vi "Fetch Multiple Records_20230203.vi"(0 "device session in":refnum<class "Device Session.lvclass">, 1 "starting record":u64, 2 "number of records":u64=1, 3 "Chan#":T1=enum."1", 5 "fetch relative to":T2=enum."First Pretrigger Sample", 7 "number of samples":u64=1000, 9 "timeout (ms)":i32=1000, 11 "error in":errorcluster, 12 "fetch offset":i64) -> (4 "device session out":refnum<class "Device Session.lvclass">, 6 "data":dbl[][](array[numeric]), 8 "relativeX (samples)":dbl[](array[numeric]), 14 "requested records info":T3[](array[typedef]), 15 "error out":errorcluster)   [LabVIEW 2021, in "Device Session.lvclass"]
doc: "Fetches data from multiple records in an acquisition. No data is returned if this VI times out. You must run the <B>Initiate</B> VI before running this VI.\n\n<B>Input Parameters</B>\n\n<B>device session in</B> is a reference to the Device Session object, which contains a session to each instrument design library used in this sample project. This parameter is obtained from the 'Open Session' VI.\n\n<B>number of records</B> specifies the number of records to fetch samples from. The default value is 1.\n\n<B>starting record</B> specifies the record to retrieve. Index of the record numbers starts at 0.\n\n<B>fetch relative to</B> specifies the relative location within the acquired record from where the VI begins to fetch data.\n\n'First Sample': the fetch starts at the first sample acquired by the device. If the device wraps data in its memory buffer, the first sample is no longer available. In this case, the VI returns an error if 'fetch offset' specifies a location that is within the overwritten portion of the memory buffer.\n'Reference Trigger Sample': the fetch starts relative to the Reference Trigger.\n'First Pretrigger Sample': the fetch starts relative to the first pretrigger sample acquired. If you do not configure a Reference Trigger, 'First Pretrigger Sample' behaves the same as 'First Sample' because there are no pretrigger samples.\n'Most Recent Sample': the fetch starts relative to the most recently acquired sample. The value of 'fetch offset' must be negative. This VI doesn't support this option. Consider using the 'Fetch Single Record' VI instead.\n'Current Read Position': the fetch starts after the last fetched sample. This VI doesn't support this option. Consider using the 'Fetch Single Record' VI instead.\n\n<B>number of samples</B> specifies the number of samples to fetch. The default value is 1000.\n\n<B>timeout (ms)</B> specifies the time, in milliseconds, allotted for the Fetch Multiple Records VI to complete execution of each record before returning a timeout error. A value of -1 specifies that the VI waits until all data is available. A value of 0 is not supported. The default value is 10,000. You cannot abort a pending fetch using the Abort VI or Close VI.\n\n<B>fetch offset</B> specifies the offset relative to the position, which is specified by the 'fetch relative to' parameter, from which to start fetching data. Offset can be a positive or negative value. The default value is 0.\n\n<B>error in</B> describes error conditions that occur before this node runs. This input provides standard 'error in' functionality.\n\n<B>Output Parameters</B>\n\n<B>device session out</B> passes a reference to the session to the next VI.\n\n<B>data</B> returns the acquired records. Each waveform corresponds to a record. If the fetch contains multiple channels, all waveforms for a record are returned before proceeding to the next record. For example, a two-channel, two-record acquisition returns four waveforms:\narray index 0 = Channel0 Record0\narray index 1 = Channel1 Record0\narray index 2 = Channel0 Record1\narray index 3 = Channel1 Record1\n\n<B>relativeX (samples)</B> returns the relative positions from the trigger to the first sample in the acquired data.\n\n<B>requested records info</B> returns additional information about each record returned by 'data'. There is one element in the 'requested records info' array for each record.\n\n<B>requested records info.number of samples</B> returns the number of samples in the record.\n\n<B>requested records info.starting sample number</B> returns the sample number of the first sample in the returned record data. Sample numbers are zero-based. Sample numbers start at zero for each record and increment by one for each acquired sample.\n\n<B>requested records info.number of channels</B> returns the number of channels in the record data.\n\n<B>requested records info.timestamps</B> returns the timestamp values that were captured for the record.\n\n<B>error out</B> contains error information. This output provides standard 'error out' functionality."
uses:
  Device Session.lvclass
  <instrlib>/_niInstr/Multirecord Acquisition/Interface/v1/Host/Public/Requested Record Info.ctl
  <instrlib>/_niInstr/Multirecord Acquisition/Interface/v1/Host/Public/Fetch Relative To Enum.ctl
  Enums/Channel Numbers.ctl
  Device Session.lvclass/Device Session.ctl
  <instrlib>/_niInstr/Multirecord Acquisition/Interface/v1/Host/Private/Fetch Multiple Records DBL Wrapper.vi
  <instrlib>/HSAI-RIO/Config/Group A/v1/Host/Main/niHSAI Group A Config v1 Host.lvclass
  <instrlib>/_niInstr/Multirecord Acquisition/Interface/v1/Host/niInstr Multirecord Acquisition v1 Host.lvclass
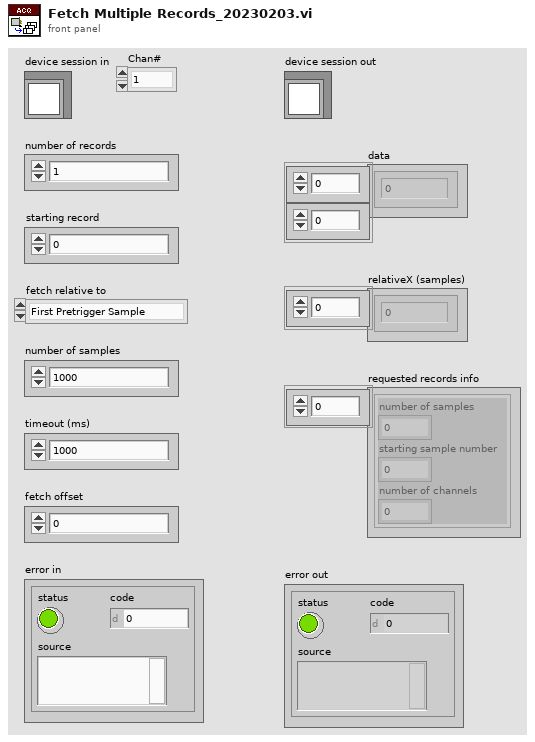
[diagram p1: front panel]
types:
  T1 = typedef "Channel Numbers.ctl" = enum16{"0", "1", "2", "3", "4", "5", "6", "7"}
  T2 = typedef "niInstr Multirecord Acquisition v1 Host.lvclass/Fetch Relative To Enum.ctl" = enum16{"First Sample", "Reference Trigger Sample", "First Pretrigger Sample", "Most Recent Sample", "Current Read Position"}
  T3 = typedef "niInstr Multirecord Acquisition v1 Host.lvclass/Requested Record Info.ctl" = cluster{"number of samples":u64, "starting sample number":u64, "number of channels":u64, "timestamps":u64[]}
  T4 = typedef "Device Session.lvclass/Device Session Object.ctl" = cluster{"fpga reference":T5, "reg bus":refnum<class "niInstr FIFO Register Bus v1 Host.lvclass">, "subsystem map":refnum<class "niInstr Subsystem Map v1 Host.lvclass">, "cal data":refnum<class "niHSAI Cal Data v1 Host.lvclass">, "config":refnum<class "niHSAI Group A Config v1 Host.lvclass">, "acquisition 0":refnum<class "niInstr Multirecord Acquisition v1 Host.lvclass">, "acquisition 1":refnum<class "niInstr Multirecord Acquisition v1 Host.lvclass">, "acquisition 2":refnum<class "niInstr Multirecord Acquisition v1 Host.lvclass">, "acquisition 3":refnum<class "niInstr Multirecord Acquisition v1 Host.lvclass">, "acquisition 4":refnum<class "niInstr Multirecord Acquisition v1 Host.lvclass">, "acquisition 5":refnum<class "niInstr Multirecord Acquisition v1 Host.lvclass">, "acquisition 6":refnum<class "niInstr Multirecord Acquisition v1 Host.lvclass">, "acquisition 7":refnum<class "niInstr Multirecord Acquisition v1 Host.lvclass">, "number of selected acq channels":u8, "selected acq channels":bool[], "number of channels":u32, "configured channels":bool[], "acq configuration":cluster{"number of samples":u64, "number of records":u64, "pretrigger samples":u64}, "actual channel configuration":T6[], "sample clock rate (Hz)":dbl, "scaling coefficients":T10[]}
  T5 = typedef "Device Session.lvclass/FPGA Refnum.ctl" = refnum<k20>
  T6 = typedef "niHSAI Types v1 Host.lvlib/Channel Configuration.ctl" = cluster{"channel":u32, "coupling":T7, "impedance":T8, "bandwidth":T9, "vertical range":dbl, "vertical offset":dbl}
  T7 = typedef "niHSAI Types v1 Host.lvlib/Coupling.ctl" = enum8{"Default", "DC", "AC"}
  T8 = typedef "niHSAI Types v1 Host.lvlib/Impedance.ctl" = enum8{"Default", "1 mega ohm", "50 ohm"}
  T9 = typedef "niHSAI Types v1 Host.lvlib/Bandwidth.ctl" = enum8{"Default", "Full Bandwidth", "Anti-alias Filter", "150 MHz"}
  T10 = typedef "niInstr Multirecord Acquisition v1 Host.lvclass/Scaling Coefficient.ctl" = cluster{"gain":dbl, "offset":dbl}
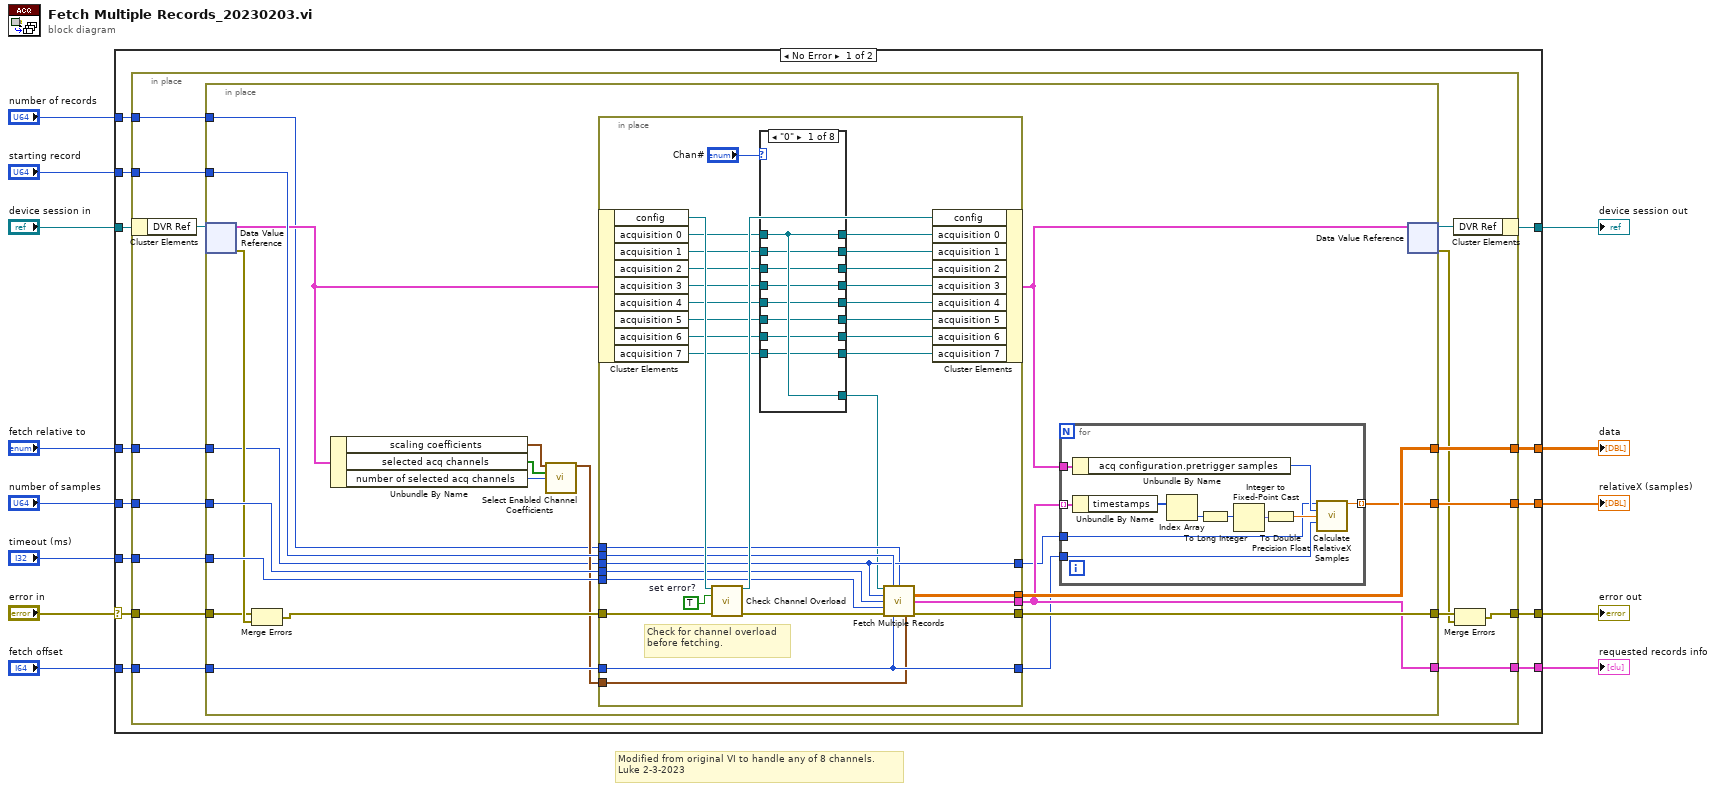
[diagram p0: block diagram]
diagram:
  # "Modified from original VI to handle any of 8 channels.\nLuke 2-3-2023"
  n1 = case shown="No Error" "error in" {
    selector: "error in" -> [w26 w172]
    tunnel: [w21 w172] -> w1
    tunnel: "device session in" -> [w16 w171]
    tunnel: [w15 w171] -> w5
    tunnel: "number of samples" -> [w25 _]
    tunnel: "timeout (ms)" -> [w24 _]
    tunnel: "fetch offset" -> [w23 _]
    tunnel: "starting record" -> [w22 _]
    tunnel: "fetch relative to" -> [w20 _]
    tunnel: [w19 _] -> w4
    tunnel: [w18 _] -> w2
    tunnel: [w17 _] -> w3
    tunnel: "number of records" -> [w14 _]
    frame No Error {
      n2 = in-place {
        in-place-border: w26 -> [w41]
        in-place-border: w25 -> [w40]
        in-place-border: w24 -> [w39]
        in-place-border: w23 -> [w38]
        in-place-border: w22 -> [w37]
        in-place-border: [w36] -> w21
        in-place-border: w20 -> [w34]
        in-place-border: [w33] -> w19
        in-place-border: [w32] -> w18
        in-place-border: [w31] -> w17
        in-place-border: w14 -> [w27]
        n3 = in-place-cluster #1(w16) -> ("DVR Ref"=w29:refnum<data-value>)
        n4 = in-place {
          in-place-border: w41 -> [w58]
          in-place-border: [w62] -> w35
          in-place-border: w40 -> [w61]
          in-place-border: w39 -> [w60]
          in-place-border: w38 -> [w50]
          in-place-border: w37 -> [w55]
          in-place-border: w34 -> [w47]
          in-place-border: [w54] -> w33
          in-place-border: [w53] -> w32
          in-place-border: [w46] -> w31
          in-place-border: w27 -> [w44]
          n5 = in-place-dvr #2(w29) -> (w48:T4, w59:errorcluster)
          n6 = Merge Errors(w58, w59) -> (w51:errorcluster)
          n7 = Unbundle By Name(w48) -> ("scaling coefficients"=w52:T10[], "selected acq channels"=w57:bool[], "number of selected acq channels"=w56:u8)
          n8 = call "Select Enabled Channel Coefficients.vi"("configured scaling coefficients"=w52, "selected acq channels to store"=w57, "number of selected acq channels to store"=w56) -> ("stored scaling coefficients"=w49:T10[])  [unwired: 12 in]
          n9 = in-place {
            in-place-border: [w106] -> w62
            in-place-border: w61 -> [w97]
            in-place-border: w60 -> [w96]
            in-place-border: w55 -> [w98]
            in-place-border: [w103] -> w54
            in-place-border: [w102] -> w46
            in-place-border: w51 -> [w101]
            in-place-border: w47 -> [w95]
            in-place-border: w50 -> [w94]
            in-place-border: w49 -> [w93]
            in-place-border: [w95] -> w43
            in-place-border: [w94] -> w42
            in-place-border: w44 -> [w92]
            w104 = TRUE  # set error?
            # "Check for channel overload before fetching."
            n10 = in-place-cluster #3(w48) -> ("config"=w100:refnum<class "niHSAI Group A Config v1 Host.lvclass">, "acquisition 0"=w90:refnum<class "niInstr Multirecord Acquisition v1 Host.lvclass">, "acquisition 1"=w87:refnum<class "niInstr Multirecord Acquisition v1 Host.lvclass">, "acquisition 2"=w86:refnum<class "niInstr Multirecord Acquisition v1 Host.lvclass">, "acquisition 3"=w85:refnum<class "niInstr Multirecord Acquisition v1 Host.lvclass">, "acquisition 4"=w84:refnum<class "niInstr Multirecord Acquisition v1 Host.lvclass">, "acquisition 5"=w83:refnum<class "niInstr Multirecord Acquisition v1 Host.lvclass">, "acquisition 6"=w82:refnum<class "niInstr Multirecord Acquisition v1 Host.lvclass">, "acquisition 7"=w81:refnum<class "niInstr Multirecord Acquisition v1 Host.lvclass">)
            n11 = call-dynamic "Check Channel Overload.vi"("session in"=w100, "set error? (T)"=w104, "error in"=w101) -> ("session out"=w99:refnum<class "niHSAI Group A Config v1 Host.lvclass">, "error out"=w105:errorcluster)  [unwired: 10 in, 1 out]
            n12 = case shown="\"0\"" "Chan#" {
              tunnel: [w114 w122 w130 w138 w146 w154 w162 w170] -> w89
              tunnel: w90 -> [w114 w122 w130 w138 w146 w154 w162 w170]
              tunnel: [w114 w115 w123 w131 w139 w147 w155 w163] -> w88
              tunnel: [w113 w115 w129 w137 w145 w153 w161 w169] -> w80
              tunnel: w87 -> [w113 w115 w129 w137 w145 w153 w161 w169]
              tunnel: [w112 w121 w123 w136 w144 w152 w160 w168] -> w79
              tunnel: w86 -> [w112 w121 w123 w136 w144 w152 w160 w168]
              tunnel: [w111 w120 w128 w131 w143 w151 w159 w167] -> w78
              tunnel: w85 -> [w111 w120 w128 w131 w143 w151 w159 w167]
              tunnel: [w110 w119 w127 w135 w139 w150 w158 w166] -> w77
              tunnel: w84 -> [w110 w119 w127 w135 w139 w150 w158 w166]
              tunnel: [w109 w118 w126 w134 w142 w147 w157 w165] -> w76
              tunnel: w83 -> [w109 w118 w126 w134 w142 w147 w157 w165]
              tunnel: [w108 w117 w125 w133 w141 w149 w155 w164] -> w75
              tunnel: w82 -> [w108 w117 w125 w133 w141 w149 w155 w164]
              tunnel: [w107 w116 w124 w132 w140 w148 w156 w163] -> w74
              tunnel: w81 -> [w107 w116 w124 w132 w140 w148 w156 w163]
              frame "0" {
              }
              frame "1" {
              }
              frame "2" {
              }
              frame "3" {
              }
              frame "4" {
              }
              frame "5" {
              }
              frame "6" {
              }
              frame "7" {
              }
            }
            n13 = call-poly <instrlib>:"Fetch Multiple Records.vi"("session in"=w88, "starting record"=w98, "number of records"=w92, "fetch relative to"=w95, "number of samples"=w97, "timeout (ms)"=w96, "error in"=w105, "fetch offset"=w94, "scaling coefficients"=w93) -> ("data"=w103:dbl[][], "requested records info"=w102:T3[], "error out"=w106:errorcluster)  [unwired: 3 in, 1 out]
            n14 = in-place-cluster #3("config"=w99, "acquisition 0"=w89, "acquisition 1"=w80, "acquisition 2"=w79, "acquisition 3"=w78, "acquisition 4"=w77, "acquisition 5"=w76, "acquisition 6"=w75, "acquisition 7"=w74) -> (w45:T4)
          }
          n15 = for {
            tunnel: [w73] -> w53 mode=indexing
            tunnel: w46 -> [w68] mode=indexing
            tunnel: w45 -> [w66]
            tunnel: w43 -> [w64]
            tunnel: w42 -> [w63]
            n16 = Unbundle By Name(w66) -> ("acq configuration.pretrigger samples"=w65:u64)
            n17 = Unbundle By Name(w68) -> ("timestamps"=w70:u64[])
            n18 = Index Array(array=w70) -> (element=w69:u64)  [unwired: 1 in]
            n19 = To Long Integer(number=w69) -> (32bit integer=w71:i32)
            n20 = Integer to Fixed-Point Cast(integer=w71) -> (fixed-point=w72:fxp<+/-,32,5>)  [unwired: 1 in]
            n21 = To Double Precision Float(number=w72) -> (double precision float=w67:dbl)
            n22 = call "Calculate RelativeX Samples.vi"("fetch relative to"=w64, "pretrigger samples"=w65, "timestamps"=w67, "fetch offset"=w63) -> ("relativeX (samples)"=w73:dbl)  [unwired: 11 in]
          }
          n23 = in-place-dvr #2(w45) -> (w28:refnum<data-value>, w30:errorcluster)
        }
        n24 = in-place-cluster #1("DVR Ref"=w28) -> (w15:refnum<class "Device Session.lvclass">)
        n25 = Merge Errors(w35, w30) -> (w36:errorcluster)
      }
    }
    frame Error {
    }
  }
  "error out" <- w1
  "device session out" <- w5
  "requested records info" <- w3
  "data" <- w4
  "relativeX (samples)" <- w2
